vi "FGV_PSP - Mercury.vi"(4 "error in":errorcluster, 6 "Function":enum16{"write", "read"}(ring), 7 "Mercury FGV":T1) -> (0 "error out":errorcluster, 3 "Mercury FGV":T1)   [LabVIEW 2016]
uses:
  Mercury - Typedefs/Mercury FGV.ctl
  Mercury - Typedefs/Actions.ctl
  Mercury - Typedefs/Status.ctl
  Mercury - Typedefs/Targets.ctl
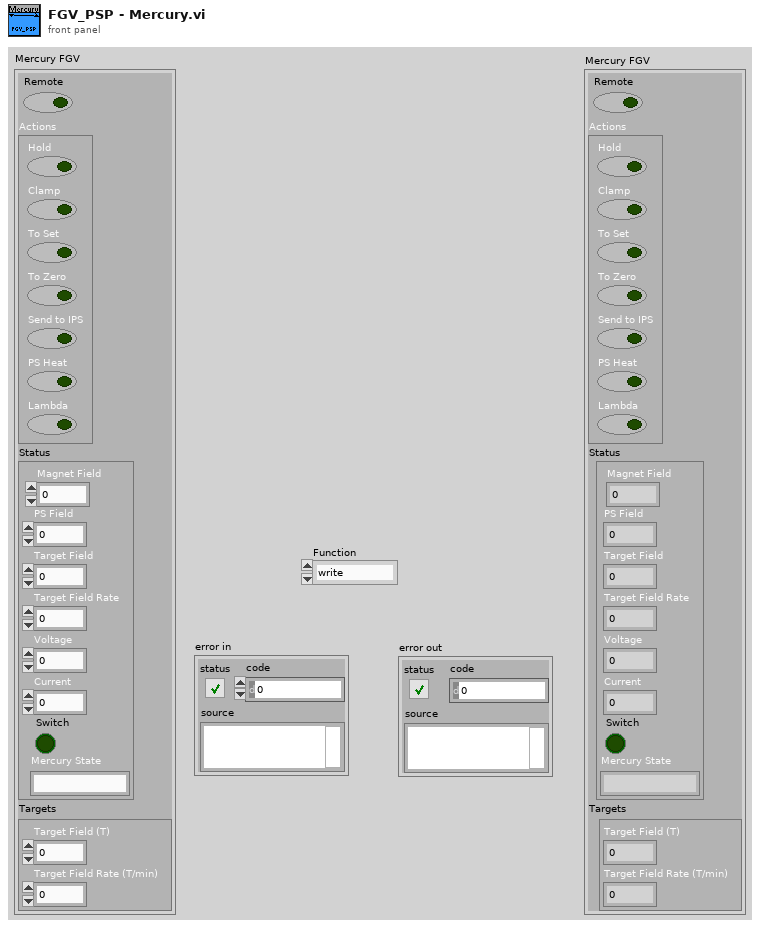
[diagram p1: front panel]
types:
  T1 = typedef "Mercury FGV.ctl" = cluster{"Remote":bool, "Actions":T2, "Status":T3, "Targets":T4}
  T2 = typedef "Actions.ctl" = cluster{"Hold":bool, "Clamp":bool, "To Set":bool, "To Zero":bool, "Send to IPS":bool, "PS Heat":bool, "Lambda":bool}
  T3 = typedef "Status.ctl" = cluster{"Magnet Field":dbl, "PS Field":dbl, "Target Field":dbl, "Target Field Rate":dbl, "Voltage":dbl, "Current":dbl, "Switch":bool, "Mercury State":string}
  T4 = typedef "Targets.ctl" = cluster{"Target Field (T)":dbl, "Target Field Rate (T/min)":dbl}
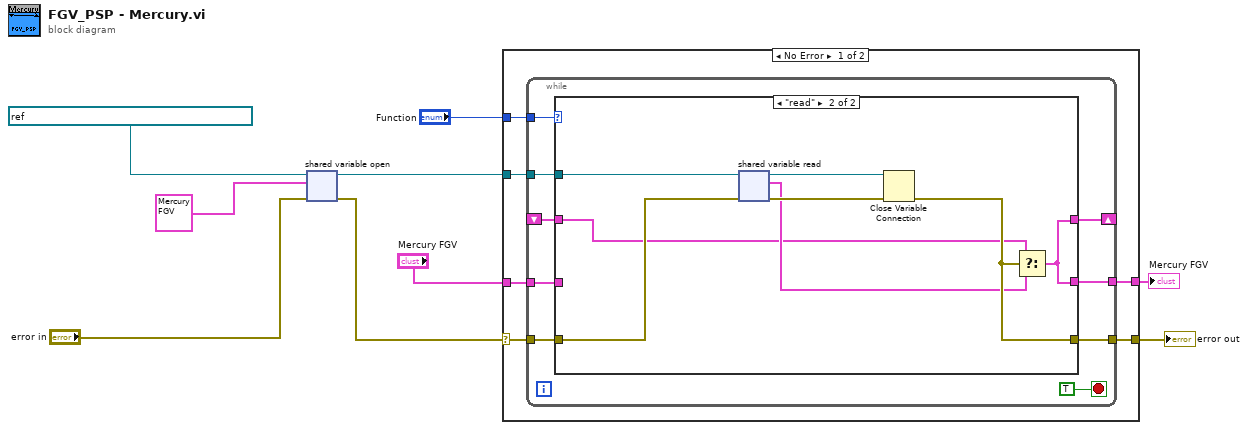
[diagram p0: block diagram]
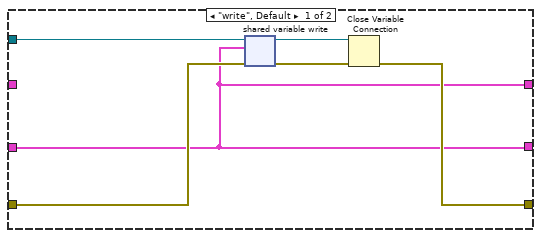
[diagram p2: hidden frame]
diagram:
  n1 = shared-variable-open(refnum<k21> "ni.var.psp://localhost/1820/Mercury" ("shared variable refnum in"), "error in", T1 {"Remote"=FALSE, "Actions"={"Hold"=FALSE, "Clamp"=FALSE, "To Set"=FALSE, "To Zero"=FALSE, "Send to IPS"=FALSE, "PS Heat"=FALSE, "Lambda"=FALSE}, "Status"={"Magnet Field"=0.0, "PS Field"=0.0, "Target Field"=0.0, "Target Field Rate"=0.0, "Voltage"=0.0, "Current"=0.0, "Switch"=FALSE, "Mercury State"=""}, "Targets"={"Target Field (T)"=0.0, "Target Field Rate (T/min)"=0.0}} ("Mercury")) -> (w7:refnum<k21>, w5:errorcluster)  [unwired: 1 in]
  n2 = case shown="No Error" w5 {
    selector: w5 -> [w15 w40]
    tunnel: [w14 w40] -> w9
    tunnel: [w13 w39] -> w1
    tunnel: "Function" -> [w12 _]
    tunnel: w7 -> [w11 _]
    tunnel: "Mercury FGV" -> [w10 w39]
    frame No Error {
      n3 = while {
        shift-right: [w19] -> _
        shift-left: _ -> [w18]
        tunnel: w15 -> [w23]
        tunnel: [w22] -> w14
        tunnel: [w21] -> w13
        tunnel: w12 -> [w20]
        tunnel: w11 -> [w17]
        tunnel: w10 -> [w16]
        stop <- TRUE stop-if-true
        n4 = case shown="\"read\"" w20 {
          tunnel: w23 -> [w27 w34]
          tunnel: [w29 w35] -> w22
          tunnel: [w25 w36] -> w21
          tunnel: [w25 w36] -> w19
          tunnel: w18 -> [_ w31]
          tunnel: w17 -> [w26 w32]
          tunnel: w16 -> [w25 _]
          frame "write", Default {
            n5 = shared-variable-write(w26, w27, w25) -> (w28:refnum<k21>, w30:errorcluster)
            n6 = Close Variable Connection(8:w30, 11:w28) -> (0:w29:errorcluster)
          }
          frame "read" {
            n7 = shared-variable-read(w32, w34) -> (w38:refnum<k21>, w37:errorcluster, w33:T1)  [unwired: 1 out]
            n8 = Close Variable Connection(8:w37, 11:w38) -> (0:w35:errorcluster)
            n9 = Select(t=w31, s=w35, f=w33) -> (s? t:f=w36:T1)
          }
        }
      }
    }
    frame Error {
    }
  }
  "error out" <- w9
  "Mercury FGV" <- w1
